vi "Periodic Tasks.vi"(8 "error in":errorcluster) -> ()   [LabVIEW 2020]
doc: "This VI runs in parallel to other tasks. It can contain as many user-defined periodic loops as you need. These can carry out PID or other sorts of timed response."
uses:
  <vilib>/Rock Robotics/WPI/Utilities/WPI_GetSetVariantRefNum.vi
panel:
  out "proximity 2":dbl
  out "B 2":dbl
  out "G 2":dbl
  out "R 2":dbl
  out "proximity":dbl
  out "B":dbl
  out "G":dbl
  out "R":dbl
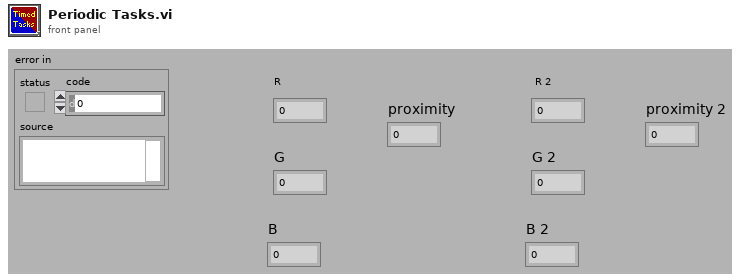
[diagram p1: front panel]
types:
  T1 = typedef "WPI_JoystickDevRef.ctl" = cluster{"Device":T2}
  T2 = typedef "WPI_JoystickDeviceEnum.ctl" = enum16{"USB 0", "USB 1", "USB 2", "USB 3", "USB 4", "USB 5"}
  T3 = typedef "WPI_RobotDriveDevRef.ctl" = cluster{"DevStatus":errorcluster, "Motors[]":T4[], "Square Inputs":bool, "Max Output":dbl}
  T4 = typedef "WPI_MotorControlDeviceRef.ctl" = cluster{"DeviceStatus":errorcluster, "Type":T5, "PWM":cluster{"PWM Channel":T6, "DeadBand":T7}, "CAN":cluster{"Device Number":u8, "SetOutput VI Ref":variant, "GetOutput VI Ref":variant, "Enable VI Ref":variant, "Disable VI Ref":variant, "Data":variant}, "Invert":bool, "DIO PWM":cluster{"PWM \"Enable\" Channel":T6, "DIOChannel":T8, "PWM Rate":dbl}}
  T5 = typedef "WPI_MotorControlType.ctl" = enum16{"PWM", "CAN", "DIO PWM"}
  T6 = typedef "FPGA_DIOPWMChannel.ctl" = enum8{"PWM 0", "PWM 1", "PWM 2", "PWM 3", "PWM 4", "PWM 5", "PWM 6", "PWM 7", "PWM 8", "PWM 9", "PWM MXP 0", "PWM MXP 1", "PWM MXP 2", "PWM MXP 3", "PWM MXP 4", "PWM MXP 5", "PWM MXP 6", "PWM MXP 7", "PWM MXP 8", "PWM MXP 9", "Invalid"}
  T7 = typedef "WPI_PWMDeadband.ctl" = cluster{"Name":string, "maxPositivePwm":i32, "minPositivePwm":i32, "centerPwm":i32, "maxNegativePwm":i32, "minNegativePwm":i32, "angularRange":u16}
  T8 = typedef "FPGA_DIOChannel.ctl" = enum8{"DIO 0", "DIO 1", "DIO 2", "DIO 3", "DIO 4", "DIO 5", "DIO 6", "DIO 7", "DIO 8", "DIO 9", "DIO MXP 0", "DIO MXP 1", "DIO MXP 2", "DIO MXP 3", "DIO MXP 4", "DIO MXP 5", "DIO MXP 6", "DIO MXP 7", "DIO MXP 8", "DIO MXP 9", "DIO MXP 10", "DIO MXP 11", "DIO MXP 12", "DIO MXP 13", "DIO MXP 14", "DIO MXP 15", "SPI Port CS1", "SPI Port CS2", "SPI Port CS3", "SPI Port MISO", "SPI Port MOSI", "Invalid"}
  T9 = cluster{"JoystickDevRef":T1, "RobotDriveDevRef":T3}
  T10 = typedef "Color Sensor V3 DevRef.ctl" = cluster{"I2CDevRef":T11}
  T11 = typedef "WPI_I2CDevRef.ctl" = cluster{"DevStatus":errorcluster, "Device Address":u8, "Handle":i32, "I2C Bus":T12}
  T12 = typedef "i2c_bus.ctl" = enum16{"I2C On-Board", "I2C MXP", "Invalid"}
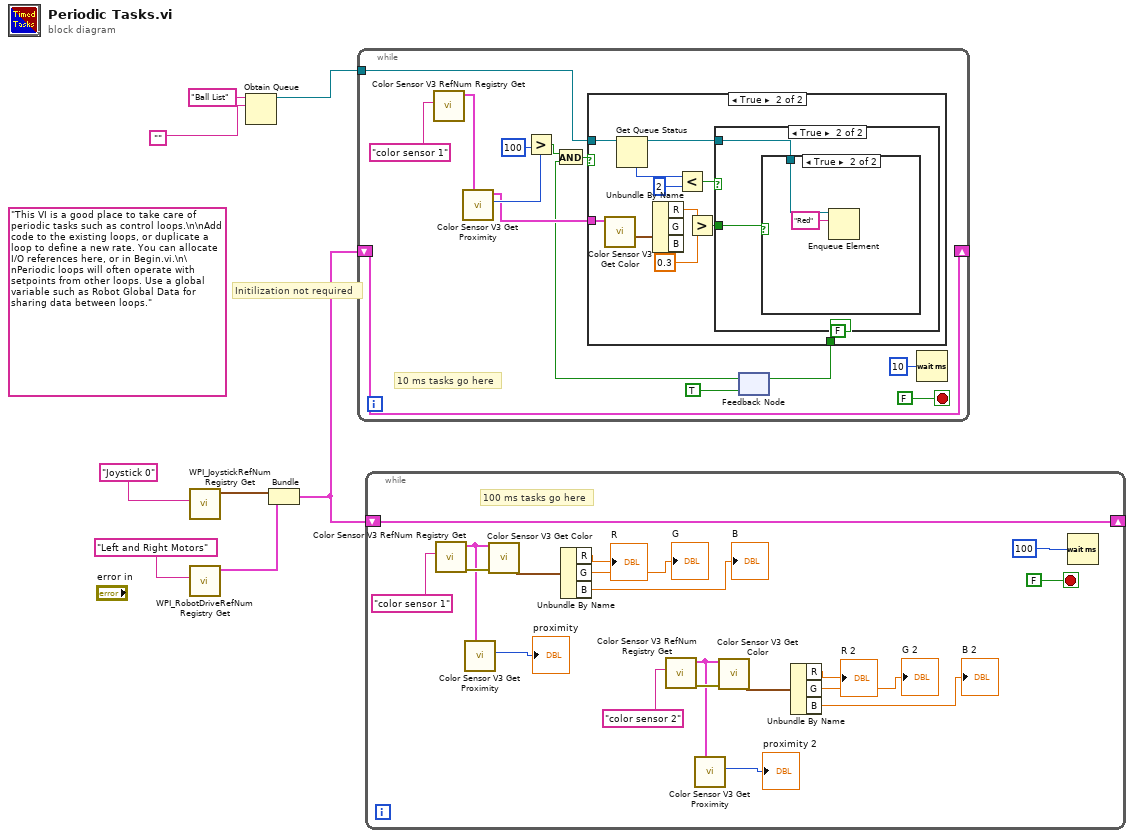
[diagram p0: block diagram]
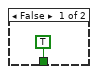
[diagram p2: hidden frame]
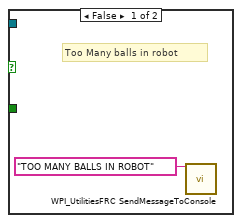
[diagram p3: hidden frame]
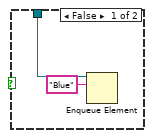
[diagram p4: hidden frame]
diagram:
  (unwired) "This VI is a good place to take care of periodic tasks such as control loops.\n\nAdd code to the existing loops, or duplicate a loop to define a new rate. You can allocate I/O references here, or in Begin.vi.\n\nPeriodic loops will often operate with setpoints from other loops. Use a global variable such as Robot Global Data for sharing data between loops."
  # "Initilization not required"
  n1 = call <vilib>:"WPI_JoystickRefNum Registry Get.vi"("refnum name"="Joystick 0") -> ("JoystickDevRef"=w6:T1)  [unwired: 1 in, 9 out]
  n2 = call <vilib>:"WPI_RobotDriveRefNum Registry Get.vi"("refnum name"="Left and Right Motors") -> ("RobotDriveDevRef"=w5:T3)  [unwired: 1 in, 9 out]
  n3 = Obtain Queue(name (unnamed)="Ball List", element data type="") -> (queue out=w3:refnum<queue>)  [unwired: 3 in, 2 out]
  n4 = Bundle("JoystickDevRef"=w6, "RobotDriveDevRef"=w5) -> (w4:T9)  [unwired: 1 out]
  n5 = while {
    shift-right: [w20] -> _
    shift-left: w4 -> [w20]
    tunnel: w3 -> [w17]
    stop <- FALSE stop-if-true
    # "10 ms tasks go here"
    n6 = call <vilib>:"Color Sensor V3 RefNum Registry Get.vi"("refnum name"="color sensor 1") -> ("ColorSensorDevRef"=w16:T10)  [unwired: 9 in, 1 out]
    n7 = call <vilib>:"Color Sensor V3 Get Proximity.vi"("ColorSensorDevRef"=w16) -> ("Proximity"=w18:u16, "ColorSensorDevRef out"=w15:T10)  [unwired: 8 in, 1 out]
    n8 = Greater?(x=u16 100, y=w18) -> (0:w13:bool)
    n9 = feedback #1(TRUE) -> (w11:bool)
    n10 = And(x=w13, y=w11) -> (x .and. y?=w12:bool)
    n11 = case shown="True" w12 {
      tunnel: w17 -> [_ w34]
      tunnel: w15 -> [_ w30]
      tunnel: [TRUE FALSE] -> w10
      frame False {
      }
      frame True {
        n12 = call <vilib>:"Color Sensor V3 Get Color.vi"("ColorSensorDevRef"=w30) -> ("Normalized Color"=w29:cluster{"R":dbl, "G":dbl, "B":dbl})  [unwired: 7 in, 3 out]
        n13 = Get Queue Status(queue=w34) -> (queue out=w25:refnum<queue>, # elements in queue=w32:i32)  [unwired: 2 in, 6 out]
        n14 = Unbundle By Name(w29) -> ("R"=w28:dbl)  [unwired: 2 out]
        n15 = Less?(x=w32, y=2) -> (x < y?=w33:bool)
        n16 = Greater?(x=w28, y=0.3) -> (0:w26:bool)
        n17 = case shown="True" w33 {
          tunnel: w26 -> [_ w37]
          tunnel: w25 -> [_ w36]
          frame False {
            # "Too Many balls in robot"
            n18 = call <vilib>:"WPI_UtilitiesFRC SendMessageToConsole.vi"("Message"="TOO MANY BALLS IN ROBOT") -> ()  [unwired: 14 in, 1 out]
          }
          frame True {
            n19 = case shown="True" w37 {
              tunnel: w36 -> [w39 w41]
              frame False {
                n20 = Enqueue Element(queue=w39, element="Blue") -> ()  [unwired: 2 in, 3 out]
              }
              frame True {
                n21 = Enqueue Element(queue=w41, element="Red") -> ()  [unwired: 2 in, 3 out]
              }
            }
          }
        }
      }
    }
    n22 = feedback-in #1(w10) -> ()
    n23 = Wait (ms)(milliseconds to wait=u32 10) -> ()  [unwired: 1 out]
  }
  n24 = while {
    shift-right: [w59] -> _
    shift-left: w4 -> [w59]
    stop <- FALSE stop-if-true
    # "100 ms tasks go here"
    n25 = call <vilib>:"Color Sensor V3 RefNum Registry Get.vi"("refnum name"="color sensor 1") -> ("error out"=w57:errorcluster, "ColorSensorDevRef"=w52:T10)  [unwired: 9 in]
    n26 = call <vilib>:"Color Sensor V3 Get Proximity.vi"("ColorSensorDevRef"=w52) -> ("Proximity"=→"proximity":u16)  [unwired: 8 in, 2 out]
    n27 = call <vilib>:"Color Sensor V3 Get Color.vi"("error in (no error)"=w57, "ColorSensorDevRef"=w52) -> ("Normalized Color"=w56:cluster{"R":dbl, "G":dbl, "B":dbl})  [unwired: 6 in, 3 out]
    n28 = Unbundle By Name(w56) -> ("R"=→"R":dbl, "G"=→"G":dbl, "B"=→"B":dbl)
    n29 = call <vilib>:"Color Sensor V3 RefNum Registry Get.vi"("refnum name"="color sensor 2") -> ("error out"=w48:errorcluster, "ColorSensorDevRef"=w43:T10)  [unwired: 9 in]
    n30 = call <vilib>:"Color Sensor V3 Get Proximity.vi"("ColorSensorDevRef"=w43) -> ("Proximity"=→"proximity 2":u16)  [unwired: 8 in, 2 out]
    n31 = call <vilib>:"Color Sensor V3 Get Color.vi"("error in (no error)"=w48, "ColorSensorDevRef"=w43) -> ("Normalized Color"=w47:cluster{"R":dbl, "G":dbl, "B":dbl})  [unwired: 6 in, 3 out]
    n32 = Unbundle By Name(w47) -> ("R"=→"R 2":dbl, "G"=→"G 2":dbl, "B"=→"B 2":dbl)
    n33 = Wait (ms)(milliseconds to wait=u32 100) -> ()  [unwired: 1 out]
  }
